vi "Read Calibration.vi"(8 "error in (no error)":errorcluster, 11 "VISA resource name":refnum<visa-resource-name>) -> (0 "error out":errorcluster, 1 "cal type":i32(ring) items=["response", "response and isolation", "S11 1-port", "S22 1-port", "full 2-port", "one path 2-port", "no cal detected"], 3 "VISA resource name out":refnum<visa-resource-name>)   [LabVIEW 2018, in "Agilent 87XX Series.lvlib"]
doc: "This VI for the HP 8753B is used to read the calibration type.\n\n0 response\n1 response and isolation\n2 S11 1-port\n3 S22 1-port\n4 full 2-port\n5 one path 2-port\n6 no cal detected"
uses:
  Agilent 87XX Series.lvlib
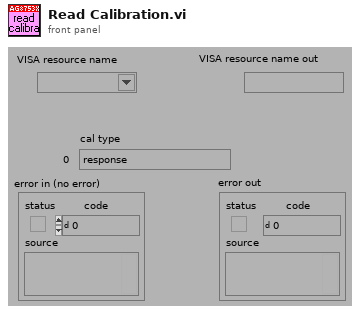
[diagram p1: front panel]
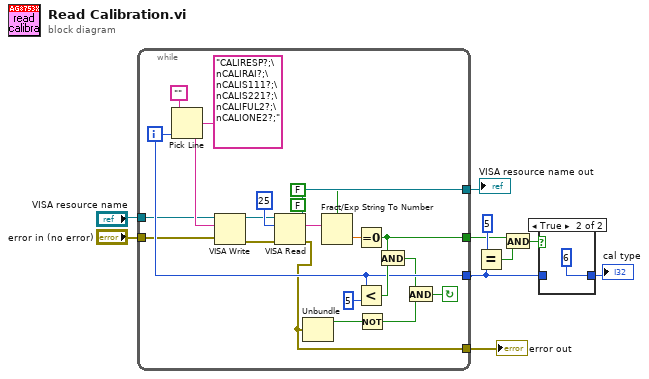
[diagram p0: block diagram]
diagram:
  n1 = while {
    tunnel: "error in (no error)" -> [w12]
    tunnel: "VISA resource name" -> [w13]
    tunnel: [w17] -> w3
    tunnel: [w14] -> w4
    tunnel: [w22] -> w5
    tunnel: [w24] -> w7
    i -> [w22]
    stop <- w18 continue-if-true
    (unwired) FALSE ("use system decimal point (T)")
    n2 = Pick Line(string ("")="", multi-line string="CALIRESP?;\nCALIRAI?;\nCALIS111?;\nCALIS221?;\nCALIFUL2?;\nCALIONE2?;", line index=w22) -> (output string=w29:string)
    n3 = VISA Write(VISA resource name=w13, write buffer=w29, error in (no error)=w12) -> (VISA resource name out=w15:refnum<visa-resource-name>, error out=w28:errorcluster)  [unwired: 1 out]
    n4 = VISA Read(VISA resource name=w15, byte count=u32 25, error in (no error)=w28) -> (VISA resource name out=w17:refnum<visa-resource-name>, read buffer=w27:string, error out=w14:errorcluster)  [unwired: 1 out]
    n5 = Unbundle(w14) -> ("status"=w21:bool)  [unwired: 2 out]
    n6 = Fract/Exp String To Number(use system decimal point (T)=FALSE, string=w27) -> (number=w26:dbl)  [unwired: 2 in, 1 out]
    n7 = Equal To 0?(x=w26) -> (x = 0?=w24:bool)
    n8 = Less?(x=w22, y=5) -> (x < y?=w23:bool)
    n9 = Not(x=w21) -> (.not. x?=w19:bool)
    n10 = And(x=w24, y=w23) -> (x .and. y?=w20:bool)
    n11 = And(x=w20, y=w19) -> (x .and. y?=w18:bool)
  }
  "VISA resource name out" <- w3
  "error out" <- w4
  n12 = Equal?(x=5, y=w5) -> (x = y?=w8:bool)
  n13 = And(x=w7, y=w8) -> (x .and. y?=w9:bool)
  n14 = case shown="True" w9 {
    tunnel: w5 -> [w32 _]
    tunnel: [w32 6] -> w6
    frame False {
    }
    frame True {
    }
  }
  "cal type" <- w6
